vi "New Verify Combinations.vi"(11 "LUnit Test Case In":refnum<class "Test Case.lvclass">) -> (0 "error out":errorcluster, 3 "LUnit Test Case Out":refnum<class "Test Case.lvclass">)   [LabVIEW 2020, in "LUnit.Extension.lvlib"]
uses:
  LUnit.Extension.lvlib
  <vilib>/Astemes/LUnit/Test Case.lvclass
  1b635337-1e38-4d08-aae1-8dabe6c40bc9.vi
  bacf86de-937c-4a87-a907-1b0971078436.vi
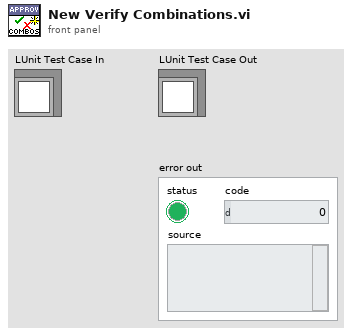
[diagram p1: front panel]
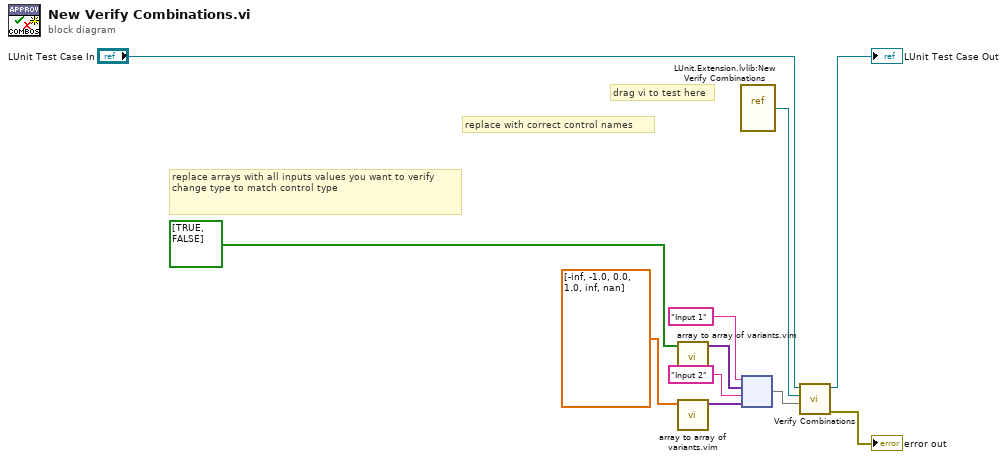
[diagram p0: block diagram]
diagram:
  # "replace arrays with all inputs values you want to verify\nchange type to match control type"
  # "replace with correct control names"
  # "drag vi to test here"
  n1 = call "array to array of variants.vim"("Array in"=bool[] [TRUE, FALSE]) -> ("Array out"=w6:variant[])  [unwired: 10 in]
  n2 = call "array to array of variants.vim"("Array in"=dbl[] [-inf, -1.0, 0.0, 1.0, inf, nan]) -> ("Array out"=w5:variant[])  [unwired: 10 in]
  n3 = vi-ref "LUnit.Extension.lvlib:New Verify Combinations.vi"() -> (w10:refnum<vi>)
  n4 = node ("Build Map")("Input 1" ("key"), w6, "Input 2" ("key"), w5) -> (w3:map{string, variant[]})
  n5 = call "Verify Combinations.vi"("ctl label -> value var[]"=w3, "VI in"=w10, "LUnit Test Case In"="LUnit Test Case In") -> ("error out"=→"error out":errorcluster, "LUnit Test Case Out"=→"LUnit Test Case Out":refnum<class "Test Case.lvclass">)  [unwired: 7 in]
